vi "Main.vi"(8 "error in (no error)":errorcluster, 11 "Galvo in vivo in":refnum<class "Galvo in vivo.lvclass">) -> (0 "error out":errorcluster, 3 "Galvo in vivo out":refnum<class "Galvo in vivo.lvclass">)   [LabVIEW 2012, in "Galvo in vivo.lvclass"]
doc: "Main VI of the component. This should contain the GUI of your component and be called when creating an executable."
uses:
  Galvo in vivo.lvclass
  <vilib>/Distrio/Murmex/Murmex/Murmex.lvclass
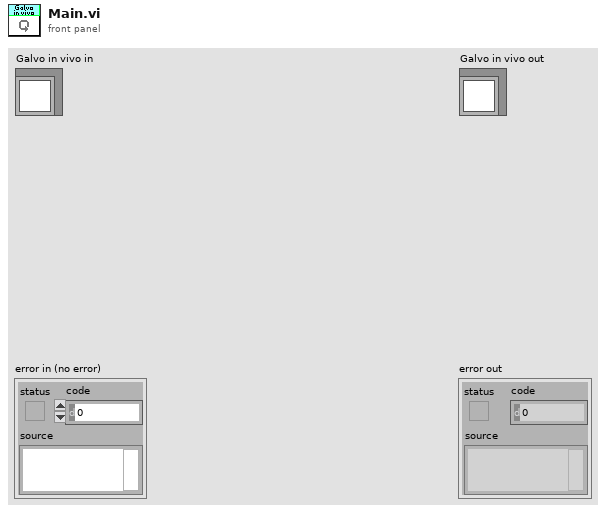
[diagram p1: front panel]
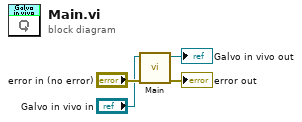
[diagram p0: block diagram]
diagram:
  n1 = call-parent "Main.vi"("error in (no error)"="error in (no error)", "Murmex in"="Galvo in vivo in") -> ("error out"=→"error out":errorcluster, "Murmex out"=→"Galvo in vivo out":refnum<class "Galvo in vivo.lvclass">)  [unwired: 8 in]
